vi "P-541 Stage Engine.vi"(0 "Notifier Name":string="SampleStageZ", 11 "COM Port":string[](array[string])) -> ()   [LabVIEW 2016]
uses:
  Stages Controls/Stage Focus Control.ctl
  Stages Controls/Stage Status.ctl
  Stages Controls/Stage Notifier Element.ctl
  Stages Controls/Stage Actions.ctl
panel:
  in  "ReInitialize":bool
  in  "Error":bool
  out "Status":T1
  in  "Quit":bool
  in  "Focus Control":T2
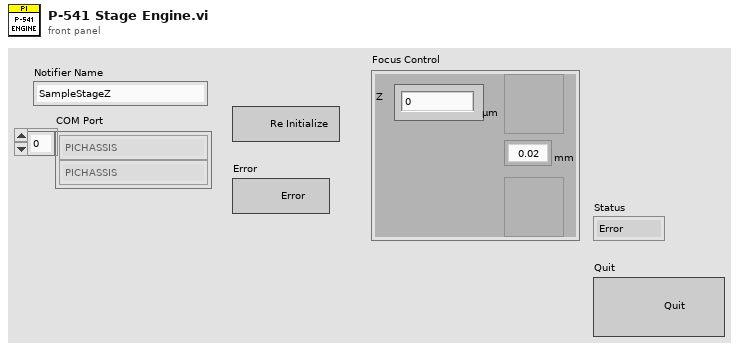
[diagram p1: front panel]
types:
  T1 = typedef "Stage Status.ctl" = enum16{"Error", "Abort", "Busy", "On Target"}
  T2 = typedef "Stage Focus Control.ctl" = cluster{"Focus Step (um)":enum16{"0.02", "0.05", "0.1", "0.5", "1", "2", "5", "10", "20"}, "Focus Up":bool, "Focus Down":bool, "Z ":dbl}
  T3 = typedef "Stage Notifier Element.ctl" = cluster{"Action":T4, "Axis":bool[], "Setpoint":dbl[], "Velocity":dbl, "Cmd Recvd?":bool, "Position":dbl[], "Status":T1, "Misc":variant}
  T4 = typedef "Stage Actions.ctl" = enum16{"Get Position", "MVR", "MOVE", "HALT", "ONTARGET", "ERROR", "REFERENCE", "INIT", "VELOCITY", "STATUS", "EXIT", "HOME", "ZEROPOS", "NANOPOS", "ANALOG", "QUIT"}
  T5 = cluster{"Focus Step (um)":bool, "Focus Up":bool, "Focus Down":bool, "Z ":bool}
  T6 = enum16{"0.02", "0.05", "0.1", "0.5", "1", "2", "5", "10", "20"}
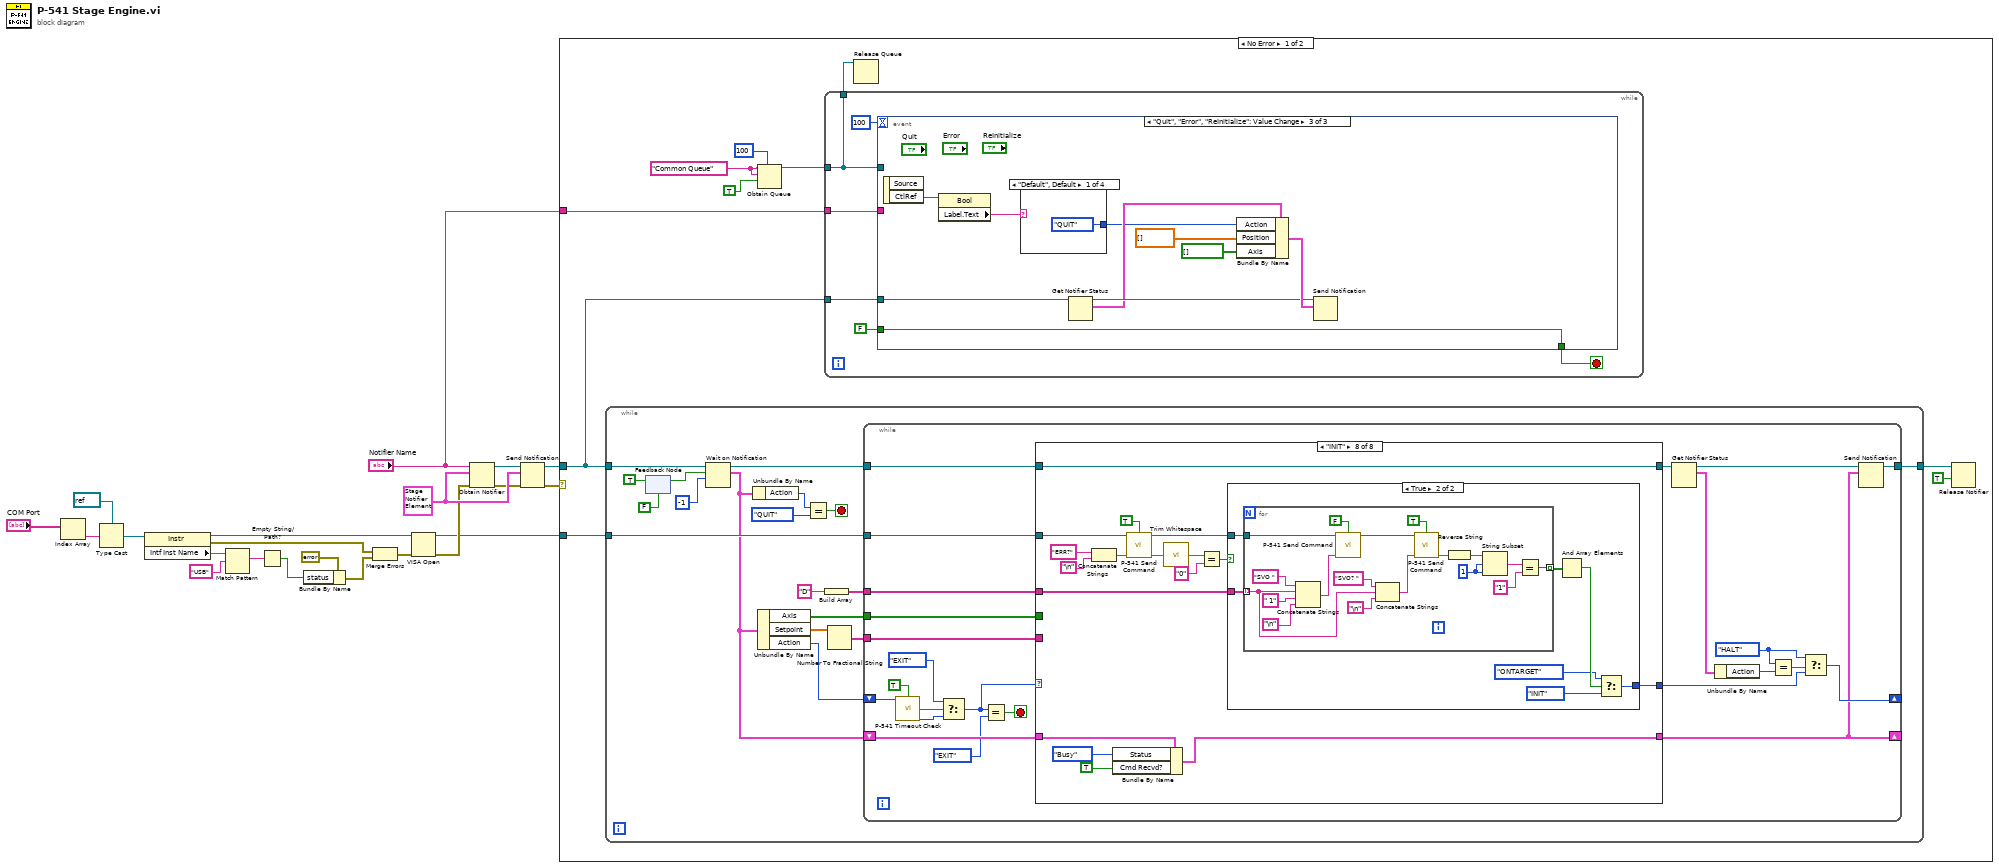
[diagram p0: block diagram]
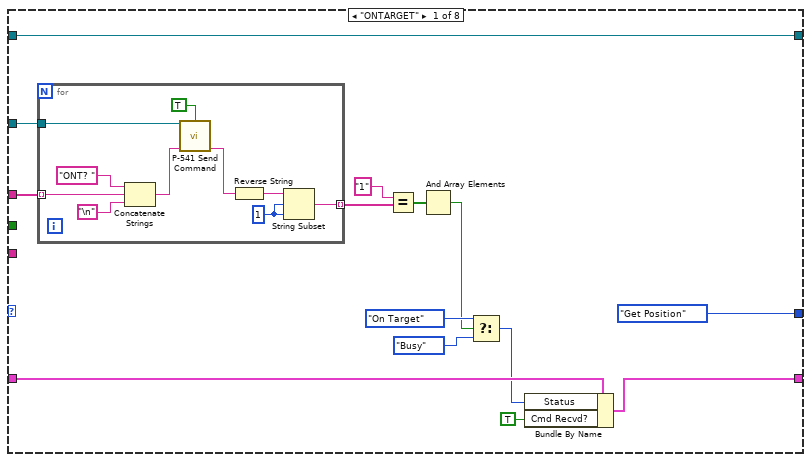
[diagram p2: hidden frame]
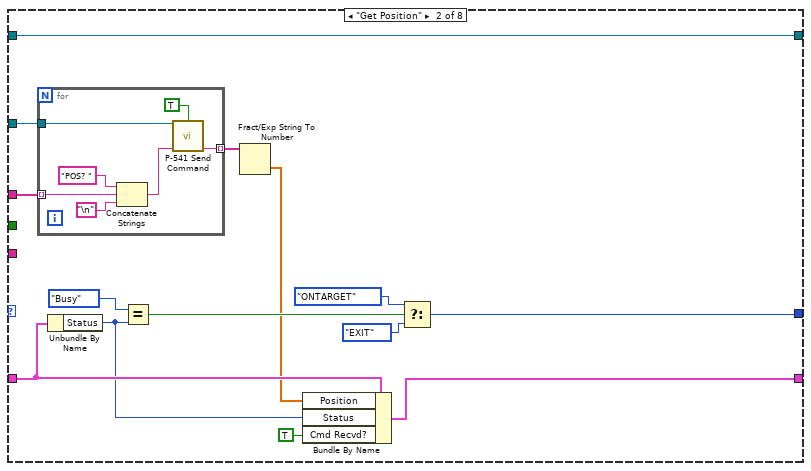
[diagram p3: hidden frame]
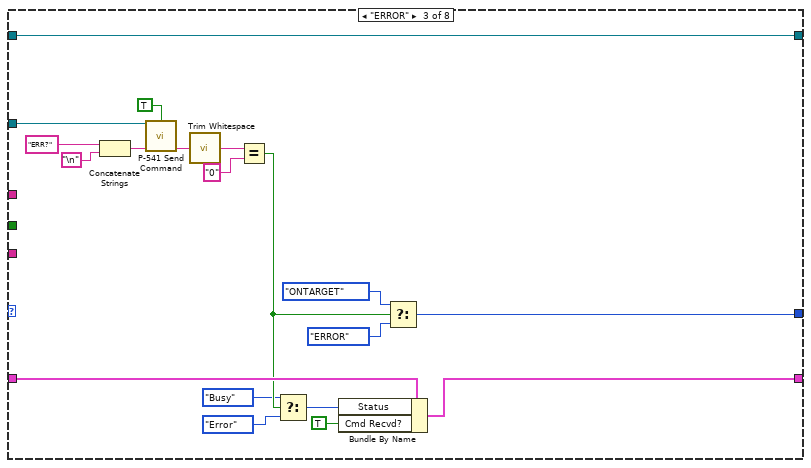
[diagram p4: hidden frame]
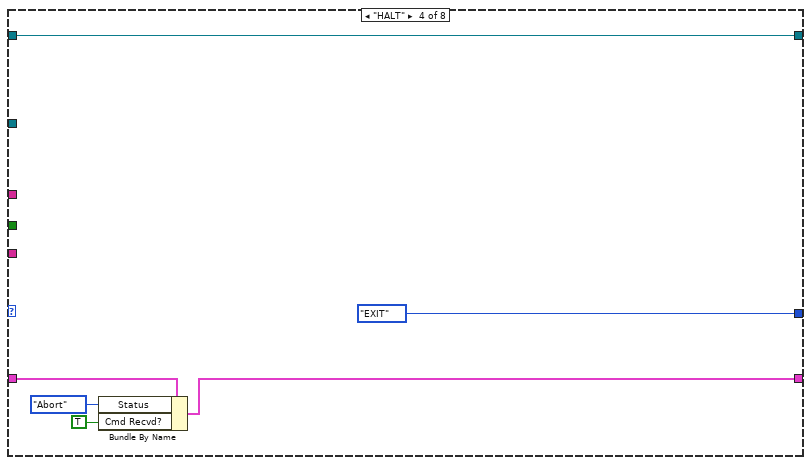
[diagram p5: hidden frame]
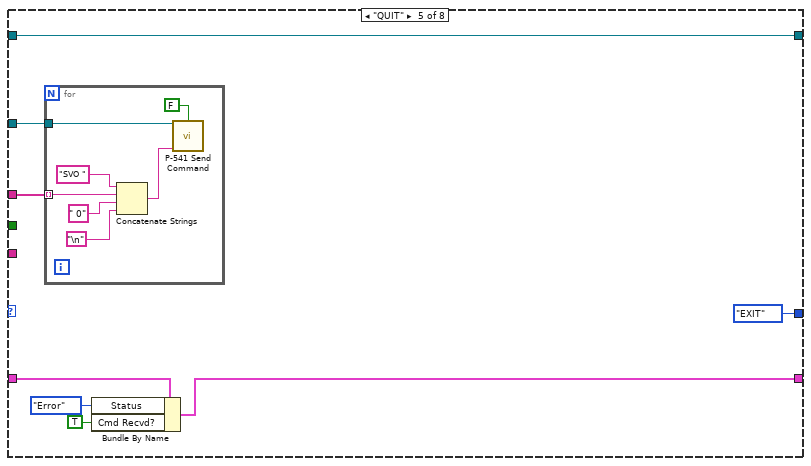
[diagram p6: hidden frame]
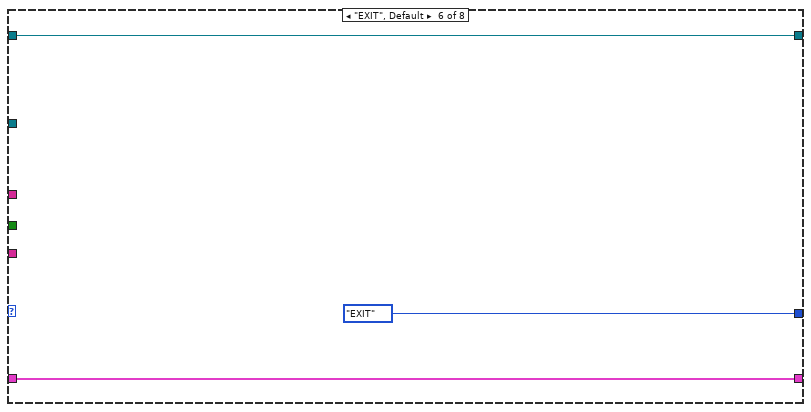
[diagram p7: hidden frame]
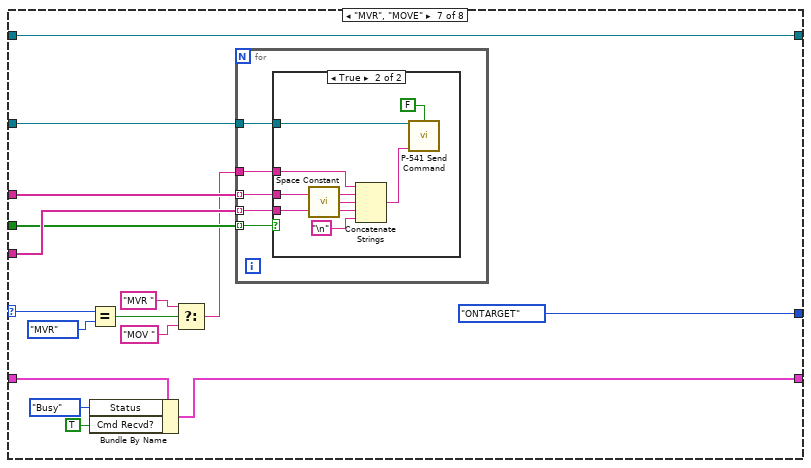
[diagram p8: hidden frame]
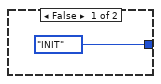
[diagram p10: hidden frame]
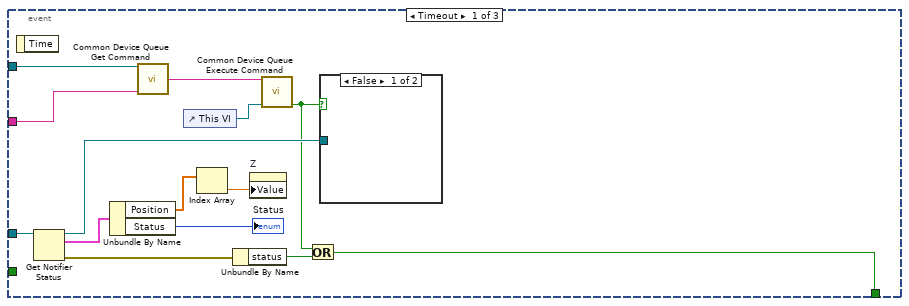
[diagram p11: hidden frame]
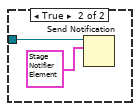
[diagram p12: hidden frame]
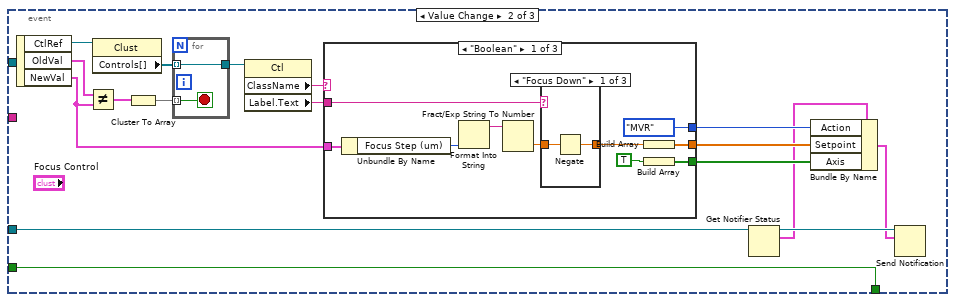
[diagram p13: hidden frame]
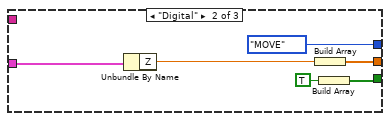
[diagram p16: hidden frame]
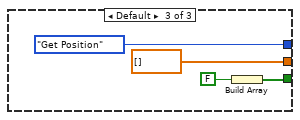
[diagram p17: hidden frame]
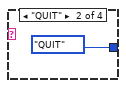
[diagram p18: hidden frame]
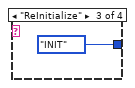
[diagram p19: hidden frame]
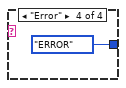
[diagram p20: hidden frame]
diagram:
  w7 = T3 {"Action"=enum."INIT", "Axis"=[], "Setpoint"=[], "Velocity"=0.5, "Cmd Recvd?"=FALSE, "Position"=[], "Status"=enum."Busy", "Misc"=variant} ("Stage Status")
  n1 = Index Array(array="COM Port") -> (element=w15:string)  [unwired: 1 in]
  n2 = Type Cast(type=refnum<visa-resource-name> refnum ("reference out"), x=w15) -> (*(type *) &x=w13:refnum<visa-resource-name>)
  n3 = property class="Instr"(reference=w13) -> (reference out=w10:refnum<visa-resource-name>, error out=w17:errorcluster, "Intf Inst Name"=w19:string)  [unwired: 1 in]
  n4 = Match Pattern(string=w19, regular expression="USB") -> (match substring=w21:string)  [unwired: 1 in, 3 out]
  n5 = Empty String/Path?(string/path=w21) -> (empty?=w18:bool)
  n6 = Bundle By Name(cluster=errorcluster {"status"=FALSE, "code"=0, "source"=""} ("Error"), "status"=w18) -> (w11:errorcluster)
  n7 = Merge Errors(w17, w11) -> (w9:errorcluster)
  n8 = VISA Open(error in (no error)=w9, VISA resource name=w10) -> (VISA resource name=w2:refnum<visa-resource-name>, error out=w5:errorcluster)  [unwired: 3 in]
  n9 = Obtain Notifier(name (unnamed)="Notifier Name", notification data type=w7, error in (no error)=w5) -> (notifier out=w8:refnum<notifier>, error out=w6:errorcluster)  [unwired: 1 in, 1 out]
  n10 = Send Notification(notification=w7, notifier=w8, error in (no error)=w6) -> (notifier out=w3:refnum<notifier>, error out=w4:errorcluster)
  n11 = case shown="No Error" w4 {
    selector: w4 -> [_ w313]
    tunnel: w3 -> [w25 w315]
    tunnel: w2 -> [w26 w314]
    tunnel: "Notifier Name" -> [w24 _]
    frame No Error {
      w29 = "Common Queue" ("Unique Notifier Name")
      n12 = while {
        tunnel: w25 -> [w48]
        tunnel: w26 -> [w39]
        tunnel: [w32] -> w22
        stop <- w49 stop-if-true
        n13 = feedback #1(FALSE) -> (w33:bool)
        n14 = feedback-in #1(TRUE) -> ()
        n15 = Wait on Notification(notifier=w48, ignore previous (F)=w33, timeout in ms (-1)=-1) -> (notifier out=w38:refnum<notifier>, notification=w37:T3)  [unwired: 1 in, 2 out]
        n16 = Unbundle By Name(w37) -> ("Action"=w47:T4)
        n17 = Unbundle By Name(w37) -> ("Axis"=w43:bool[], "Setpoint"=w44:dbl[], "Action"=w45:T4)
        n18 = Equal?(x=w47, y=Stage_Actions."QUIT") -> (x = y?=w49:bool)
        n19 = Build Array("D") -> (w41:string[])
        n20 = Number To Fractional String(number=w44) -> (F-format string=w42:string[])  [unwired: 3 in]
        n21 = while {
          tunnel: w41 -> [w73]
          shift-right: [w54] -> _
          shift-left: w45 -> [w65]
          tunnel: w43 -> [w70]
          tunnel: w42 -> [w71]
          shift-right: [w53] -> _
          shift-left: w37 -> [w69]
          tunnel: w39 -> [w72]
          tunnel: w38 -> [w51]
          tunnel: [w50] -> w32
          stop <- w67 stop-if-true
          w56 = Stage_Actions."HALT" ("Action")
          n22 = call "P-541 Timeout Check.vi"("Action"=w65, "User Input?"=TRUE) -> ("Timeout?"=w64:bool, "Action (Dup)"=w63:T4)  [unwired: 12 in]
          n23 = Select(t=Stage_Actions."EXIT" ("y"), s=w64, f=w63) -> (s? t:f=w61:T4)
          n24 = Equal?(x=w61, y=Stage_Actions."EXIT") -> (x = y?=w67:bool)
          n25 = case shown="\"INIT\"" w61 {
            selector: w61 -> [_ _ _ _ _ _ w168 _]
            tunnel: w73 -> [w87 w111 _ _ w149 _ w177 w207]
            tunnel: w72 -> [w83 w110 w123 _ w150 _ w176 w195]
            tunnel: w71 -> [_ _ _ _ _ _ w175 _]
            tunnel: w70 -> [_ _ _ _ _ _ w174 _]
            tunnel: [Stage_Actions."Get Position" ("y") w108 w132 Stage_Actions."EXIT" ("y") Stage_Actions."EXIT" ("y") Stage_Actions."EXIT" ("y") Stage_Actions."ONTARGET" ("y") w203] -> w55
            tunnel: w69 -> [w80 w106 w127 w139 w147 w161 w171 w204]
            tunnel: [w81 w103 w128 w140 w145 w161 w170 w197] -> w53
            tunnel: [w74 w98 w119 w138 w144 w159 w162 w191] -> w52
            tunnel: w51 -> [w74 w98 w119 w138 w144 w159 w162 w191]
            frame "ONTARGET" {
              n26 = for {
                tunnel: w87 -> [w97] mode=indexing
                tunnel: [w96] -> w86 mode=indexing
                tunnel: w83 -> [w90]
                w92 = 1 ("length (rest)")
                n27 = Concatenate Strings("ONT? " ("string"), w97, "\n") -> (w89:string)
                n28 = call "P-541 Send Command.vi"("VISA Ref"=w90, "Wait for Reply?"=TRUE, "Command"=w89) -> ("Response"=w88:string)  [unwired: 10 in, 2 out]
                n29 = Reverse String(1:w88) -> (0:w93:string)
                n30 = String Subset(string=w93, offset (0)=w92, length (rest)=w92) -> (substring=w96:string)
              }
              n31 = Equal?(x="1", y=w86) -> (x = y?=w84:bool[])
              n32 = And Array Elements(Boolean array=w84) -> (logical AND=w77:bool)
              n33 = Select(t=Stage_Status."On Target" ("Status"), s=w77, f=Stage_Status."Busy" ("Status")) -> (s? t:f=w76:T1)
              n34 = Bundle By Name(cluster=w80, "Status"=w76, "Cmd Recvd?"=TRUE) -> (w81:T3)
            }
            frame "Get Position" {
              n35 = for {
                tunnel: w111 -> [w118] mode=indexing
                tunnel: w110 -> [w114]
                tunnel: [w112] -> w109 mode=indexing
                n36 = Concatenate Strings("POS? " ("string"), w118, "\n") -> (w113:string)
                n37 = call "P-541 Send Command.vi"("VISA Ref"=w114, "Wait for Reply?"=TRUE, "Command"=w113) -> ("Response"=w112:string)  [unwired: 10 in, 2 out]
              }
              n38 = Unbundle By Name(w106) -> ("Status"=w101:T1)
              n39 = Equal?(x=Stage_Status."Busy", y=w101) -> (x = y?=w104:bool)
              n40 = Fract/Exp String To Number(string=w109) -> (number=w102:dbl[])  [unwired: 3 in, 1 out]
              n41 = Bundle By Name(cluster=w106, "Position"=w102, "Status"=w101, "Cmd Recvd?"=TRUE) -> (w103:T3)
              n42 = Select(t=Stage_Actions."ONTARGET" ("y"), s=w104, f=Stage_Actions."EXIT" ("y")) -> (s? t:f=w108:T4)
            }
            frame "ERROR" {
              n43 = Concatenate Strings("ERR?" ("string"), "\n") -> (w122:string)
              n44 = call "P-541 Send Command.vi"("VISA Ref"=w123, "Wait for Reply?"=TRUE, "Command"=w122) -> ("Response"=w121:string)  [unwired: 10 in, 2 out]
              n45 = call <vilib>:"Trim Whitespace.vi"("string"=w121) -> ("trimmed string"=w137:string)  [unwired: 1 in]
              n46 = Equal?(x=w137, y="0") -> (x = y?=w126:bool)
              n47 = Select(t=Stage_Status."Busy" ("Status"), s=w126, f=Stage_Status."Error" ("Status")) -> (s? t:f=w130:T1)
              n48 = Bundle By Name(cluster=w127, "Status"=w130, "Cmd Recvd?"=TRUE) -> (w128:T3)
              n49 = Select(t=Stage_Actions."ONTARGET" ("Action"), s=w126, f=Stage_Actions."ERROR") -> (s? t:f=w132:T4)
            }
            frame "HALT" {
              n50 = Bundle By Name(cluster=w139, "Status"=Stage_Status."Abort", "Cmd Recvd?"=TRUE) -> (w140:T3)
            }
            frame "QUIT" {
              n51 = for {
                tunnel: w149 -> [w155] mode=indexing
                tunnel: w150 -> [w153]
                n52 = Concatenate Strings("SVO " ("write buffer"), w155, " 0" ("string"), "\n") -> (w152:string)
                n53 = call "P-541 Send Command.vi"("VISA Ref"=w153, "Wait for Reply?"=FALSE, "Command"=w152) -> ()  [unwired: 10 in, 3 out]
              }
              n54 = Bundle By Name(cluster=w147, "Status"=Stage_Status."Error", "Cmd Recvd?"=TRUE) -> (w145:T3)
            }
            frame "EXIT", Default {
            }
            frame "MVR", "MOVE" {
              n55 = Equal?(x=w168, y=Stage_Actions."MVR") -> (x = y?=w166:bool)
              n56 = Bundle By Name(cluster=w171, "Status"=Stage_Status."Busy", "Cmd Recvd?"=TRUE) -> (w170:T3)
              n57 = Select(t="MVR ", s=w166, f="MOV ") -> (s? t:f=w163:string)
              n58 = for {
                tunnel: w177 -> [w182] mode=indexing
                tunnel: w175 -> [w181] mode=indexing
                tunnel: w174 -> [w179] mode=indexing
                tunnel: w176 -> [w180]
                tunnel: w163 -> [w178]
                n59 = case shown="True" w179 {
                  tunnel: w182 -> [_ w190]
                  tunnel: w181 -> [_ w187]
                  tunnel: w180 -> [_ w185]
                  tunnel: w178 -> [_ w183]
                  frame False {
                  }
                  frame True {
                    n60 = call <vilib>:"Space Constant.vi"() -> ("String"=w188:string)
                    n61 = Concatenate Strings(w183, w190, w188, w187, "\n") -> (w184:string)
                    n62 = call "P-541 Send Command.vi"("VISA Ref"=w185, "Wait for Reply?"=FALSE, "Command"=w184) -> ()  [unwired: 10 in, 3 out]
                  }
                }
              }
            }
            frame "INIT" {
              n63 = Concatenate Strings("ERR?" ("string"), "\n") -> (w194:string)
              n64 = Bundle By Name(cluster=w204, "Status"=Stage_Status."Busy", "Cmd Recvd?"=TRUE) -> (w197:T3)
              n65 = call "P-541 Send Command.vi"("VISA Ref"=w195, "Wait for Reply?"=TRUE, "Command"=w194) -> ("VISA Ref Out"=w192:refnum<visa-resource-name>, "Response"=w193:string)  [unwired: 10 in, 1 out]
              n66 = call <vilib>:"Trim Whitespace.vi"("string"=w193) -> ("trimmed string"=w200:string)  [unwired: 1 in]
              n67 = Equal?(x=w200, y="0") -> (x = y?=w198:bool)
              n68 = case shown="True" w198 {
                tunnel: w207 -> [_ w215]
                tunnel: [Stage_Actions."INIT" ("y") w211] -> w203
                tunnel: w192 -> [_ w209]
                frame False {
                }
                frame True {
                  n69 = for {
                    tunnel: w215 -> [w226] mode=indexing
                    tunnel: [w224] -> w214 mode=indexing
                    tunnel: w209 -> [w222]
                    w233 = 1 ("length (rest)")
                    n70 = Concatenate Strings("SVO " ("string"), w226, " 1" ("string"), "\n") -> (w221:string)
                    n71 = call "P-541 Send Command.vi"("VISA Ref"=w222, "Wait for Reply?"=FALSE, "Command"=w221) -> ("VISA Ref Out"=w219:refnum<visa-resource-name>)  [unwired: 10 in, 2 out]
                    n72 = Concatenate Strings("SVO? " ("string"), w226, "\n") -> (w218:string)
                    n73 = call "P-541 Send Command.vi"("VISA Ref"=w219, "Wait for Reply?"=TRUE, "Command"=w218) -> ("Response"=w217:string)  [unwired: 10 in, 2 out]
                    n74 = Reverse String(1:w217) -> (0:w232:string)
                    n75 = String Subset(string=w232, offset (0)=w233, length (rest)=w233) -> (substring=w216:string)
                    n76 = Equal?(x=w216, y="1") -> (x = y?=w224:bool)
                  }
                  n77 = And Array Elements(Boolean array=w214) -> (logical AND=w213:bool)
                  n78 = Select(t=Stage_Actions."ONTARGET" ("y"), s=w213, f=Stage_Actions."INIT" ("y")) -> (s? t:f=w211:T4)
                }
              }
            }
          }
          n79 = Get Notifier Status(notifier=w52) -> (notifier out=w60:refnum<notifier>, current notification=w59:T3)  [unwired: 1 in, 3 out]
          n80 = Unbundle By Name(w59) -> ("Action"=w58:T4)
          n81 = Equal?(x=w56, y=w58) -> (x = y?=w57:bool)
          n82 = Select(t=w56, s=w57, f=w55) -> (s? t:f=w54:T4)
          n83 = Send Notification(notification=w53, notifier=w60) -> (notifier out=w50:refnum<notifier>)  [unwired: 1 in, 1 out]
        }
      }
      n84 = Obtain Queue(max queue size (-1, unlimited)=100, name (unnamed)=w29, element data type=w29, create if not found? (T)=TRUE) -> (queue out=w28:refnum<queue>)  [unwired: 1 in, 2 out]
      n85 = while {
        tunnel: w25 -> [w237]
        tunnel: w28 -> [w236]
        tunnel: [w236] -> w27
        tunnel: w24 -> [w235]
        stop <- w238 stop-if-true
        n86 = event shown="[2] \"Quit\", \"Error\", \"ReInitialize\": Value Change" {
          selector: _ -> [_ _ _]
          dyn-events: _ -> [_ _ _]
          timeout: 100 -> [_ _ _]
          tunnel: [w241 w256 w299] -> w238
          tunnel: w237 -> [w252 w261 w305]
          tunnel: w236 -> [w245 _ _]
          tunnel: w235 -> [w240 _ _]
          tunnel: FALSE ("create if not found? (T)") -> [_ w256 w299]
          event Timeout {
            n87 = event-data() -> ()  [unwired: 1 in, 1 out]
            n88 = Get Notifier Status(notifier=w252) -> (notifier out=w244:refnum<notifier>, current notification=w248:T3, error out=w250:errorcluster)  [unwired: 1 in, 2 out]
            n89 = Unbundle By Name(w248) -> ("Position"=w251:dbl[], "Status"=→"Status":T1)
            n90 = call "Common Device Queue Get Command.vi"("Common Queue"=w245, "Notifier Name"=w240) -> ("Command"=w246:string)  [unwired: 12 in, 1 out]
            n91 = control-ref of="This VI"() -> (w247:refnum<vi>)
            n92 = Index Array(array=w251) -> (element=w253:dbl)  [unwired: 1 in]
            n93 = Unbundle By Name(w250) -> ("status"=w243:bool)
            n94 = property on="Z" class="DigNum (strict)"("Value"=w253) -> ()  [unwired: 2 in, 2 out]
            n95 = call "Common Device Queue Execute Command.vi"("Common Command"=w246, "VI Refnum"=w247) -> ("Quit?"=w242:bool)  [unwired: 12 in, 1 out]
            n96 = Or(x=w242, y=w243) -> (x .or. y?=w241:bool)
            n97 = case shown="False" w242 {
              tunnel: w244 -> [_ w255]
              frame False {
              }
              frame True {
                n98 = Send Notification(notification=T3 {"Action"=enum."QUIT", "Axis"=[], "Setpoint"=[], "Velocity"=0.5, "Cmd Recvd?"=FALSE, "Position"=[], "Status"=enum."Error", "Misc"=variant} ("Stage Status"), notifier=w255) -> ()  [unwired: 1 in, 2 out]
              }
            }
          }
          event Value Change {
            n99 = event-data() -> ("CtlRef"=w271:refnum<vi>, "OldVal"=w272:T2, "NewVal"=w265:T2)  [unwired: 1 in]
            n100 = Not Equal?(x=w272, y=w265) -> (x != y?=w270:T5)
            n101 = property class="Clust"(reference=w271) -> ("Controls[]"=w268:refnum<vi>[])  [unwired: 1 in, 2 out]
            n102 = Cluster To Array(cluster=w270) -> (array=w269:bool[])
            n103 = for {
              tunnel: w269 -> [w298] mode=indexing
              tunnel: [w297] -> w267
              tunnel: w268 -> [w297] mode=indexing
              stop <- w298 stop-if-true
            }
            n104 = property class="Ctl"(reference=w267) -> ("ClassName"=w266:string, "Label.Text"=w264:string)  [unwired: 1 in, 2 out]
            n105 = case shown="\"Boolean\"" w266 {
              tunnel: w265 -> [w280 w292 _]
              tunnel: w264 -> [w281 _ _]
              tunnel: [w275 w290 dbl[] []] -> w263
              tunnel: [w274 w289 w295] -> w262
              tunnel: [Stage_Actions."MVR" ("Action") Stage_Actions."MOVE" ("Action") Stage_Actions."Get Position" ("Action")] -> w260
              frame "Boolean" {
                n106 = Unbundle By Name(w280) -> ("Focus Step (um)"=w278:T6)
                n107 = Format Into String(w278) -> (resulting string=w279:string)  [unwired: 3 in, 1 out]
                n108 = Fract/Exp String To Number(string=w279) -> (number=w277:dbl)  [unwired: 3 in, 1 out]
                n109 = case shown="\"Focus Down\"" w281 {
                  tunnel: w277 -> [w284 w285 w286]
                  tunnel: [w283 w285 w286] -> w276
                  frame "Focus Down" {
                    n110 = Negate(x=w284) -> (-x=w283:dbl)
                  }
                  frame "Focus Up" {
                  }
                  frame Default {
                  }
                }
                n111 = Build Array(w276) -> (w275:dbl[])
                n112 = Build Array(TRUE) -> (w274:bool[])
              }
              frame "Digital" {
                n113 = Unbundle By Name(w292) -> ("Z"=w291:dbl)
                n114 = Build Array(w291) -> (w290:dbl[])
                n115 = Build Array(TRUE) -> (w289:bool[])
              }
              frame Default {
                n116 = Build Array(FALSE) -> (w295:bool[])
              }
            }
            n117 = Get Notifier Status(notifier=w261) -> (notifier out=w259:refnum<notifier>, current notification=w258:T3)  [unwired: 1 in, 3 out]
            n118 = Bundle By Name(cluster=w258, "Action"=w260, "Setpoint"=w263, "Axis"=w262) -> (w257:T3)
            n119 = Send Notification(notification=w257, notifier=w259) -> ()  [unwired: 1 in, 2 out]
          }
          event "Quit", "Error", "ReInitialize": Value Change {
            n120 = event-data() -> ("CtlRef"=w302:refnum<vi>)  [unwired: 1 in, 1 out]
            n121 = property class="Bool"(reference=w302) -> ("Label.Text"=w301:string)  [unwired: 1 in, 2 out]
            n122 = case shown="\"Default\", Default" w301 {
              tunnel: [Stage_Actions."QUIT" ("Action") Stage_Actions."QUIT" ("Action") Stage_Actions."INIT" ("Action") Stage_Actions."ERROR" ("Action")] -> w300
              frame "Default", Default {
              }
              frame "QUIT" {
              }
              frame "ReInitialize" {
              }
              frame "Error" {
              }
            }
            n123 = Get Notifier Status(notifier=w305) -> (notifier out=w304:refnum<notifier>, current notification=w303:T3)  [unwired: 1 in, 3 out]
            n124 = Bundle By Name(cluster=w303, "Action"=w300, "Position"=dbl[] [], "Axis"=bool[] []) -> (w306:T3)
            n125 = Send Notification(notification=w306, notifier=w304) -> ()  [unwired: 1 in, 2 out]
          }
        }
      }
      n126 = Release Queue(queue=w27) -> ()  [unwired: 2 in, 3 out]
      n127 = Release Notifier(notifier=w22, force destroy? (F)=TRUE) -> ()  [unwired: 1 in, 3 out]
    }
    frame Error {
      n128 = VISA Close(VISA resource name=w314, error in (no error)=w313) -> (error out=w316:errorcluster)
      n129 = Release Notifier(notifier=w315, force destroy? (F)=TRUE, error in (no error)=w316) -> (error out=w321:errorcluster)  [unwired: 2 out]
      n130 = Unbundle By Name(w321) -> ("source"=w318:string)
      n131 = Concatenate Strings("P-541 Stage Error", "\r", w318) -> (w317:string)
      n132 = One Button Dialog(message=w317) -> ()  [unwired: 1 in, 1 out]
    }
  }
